vi "Gyro Globals.vi"() -> ()   [LabVIEW 2013]
panel:
  in  "Reset?":bool
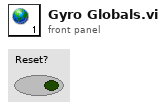
[diagram p1: front panel]
diagram:
